vi "Create and Write Header.vi"(0 "reference in":refnum<class "RPC.lvclass">, 5 "error in (no error)":errorcluster) -> (7 "Nb Channels":i32, 9 "Total Nb Samples":i32, 11 "Scaling factors":dbl[](array[numeric]), 13 "Nb Groups":i32, 14 "reference out":refnum<class "RPC.lvclass">, 19 "error out":errorcluster)   [LabVIEW 2022 SP3, in "RPC.lvclass"]
uses:
  RPC.lvclass
  API/GSwFormDSP_class/GSwFormDSP.lvclass
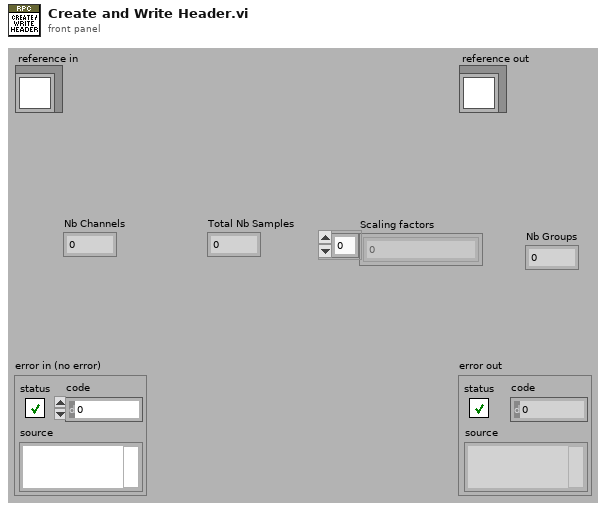
[diagram p1: front panel]
types:
  T1 = typedef "RPC.lvclass/ObjectAttributes.ctl" = cluster{"File Refnum":refnum<file>, "File total size":i32, "Offset from start of file":i32, "Time Type":enum16{"Response", "Drive"}, "Full Scale":dbl[unit], "New Time Data Obj?":bool, "Header":cluster{"Num Header":i32, "Num Parameter":i32, "Nb Channels":i32, "dT":dbl, "Number of Groups":i32, "Group size":i32, "Units":string[], "Names":string[], "Sensitivity":dbl[], "Complete header":string[]}, "Time Data":refnum<class "GSwFormDSP.lvclass">}
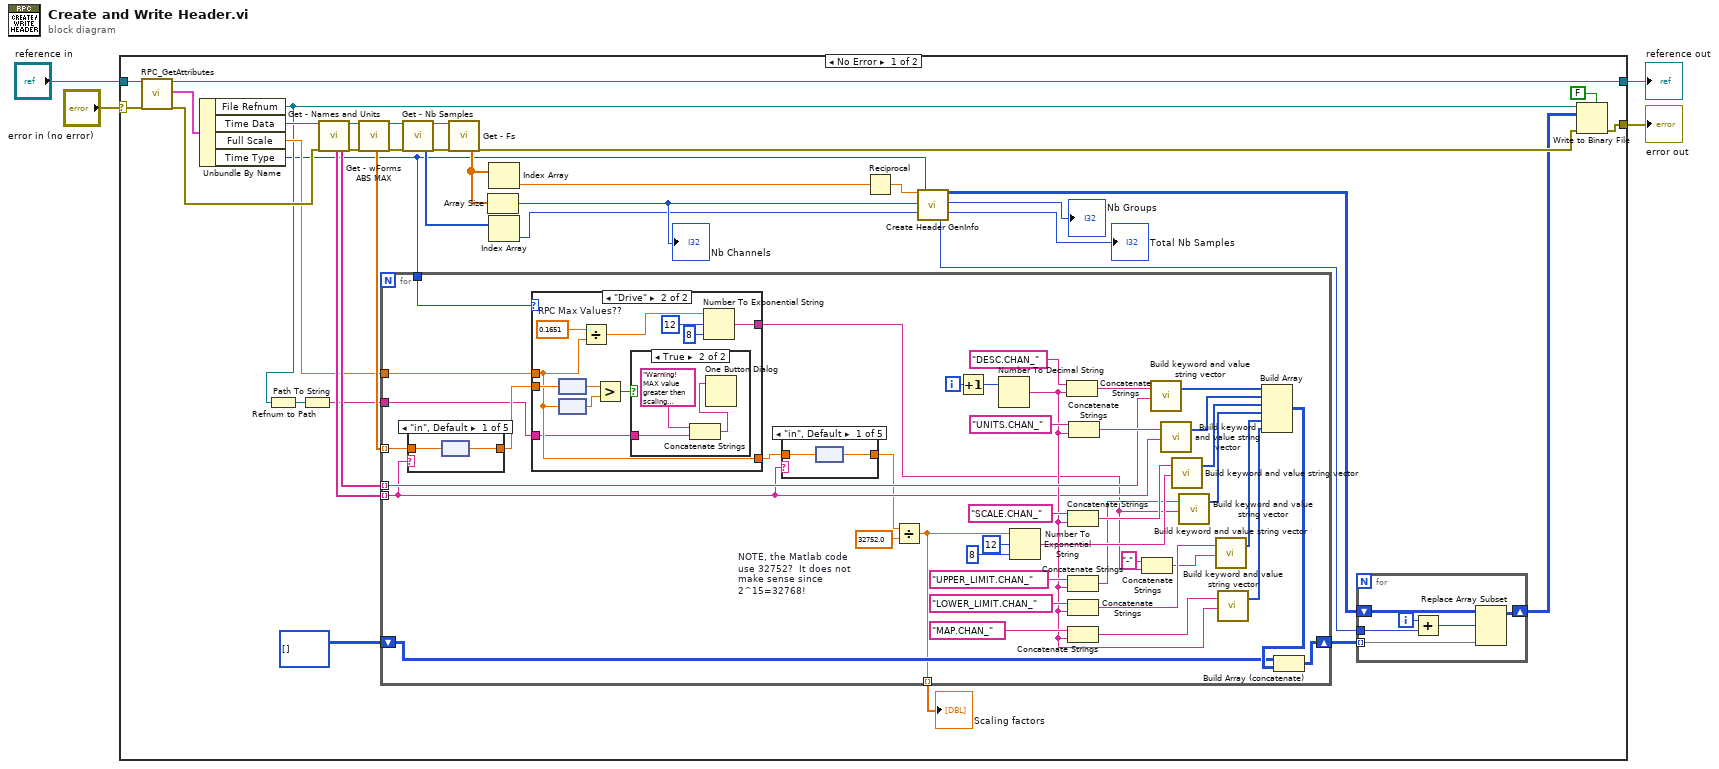
[diagram p0: block diagram]
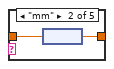
[diagram p2: hidden frame]
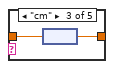
[diagram p3: hidden frame]
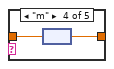
[diagram p4: hidden frame]
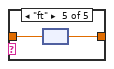
[diagram p5: hidden frame]
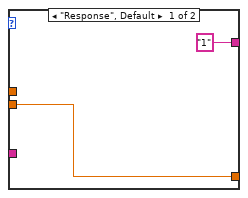
[diagram p6: hidden frame]
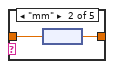
[diagram p8: hidden frame]
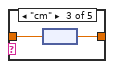
[diagram p9: hidden frame]
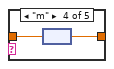
[diagram p10: hidden frame]
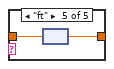
[diagram p11: hidden frame]
diagram:
  n1 = case shown="No Error" "error in (no error)" {
    selector: "error in (no error)" -> [w41 w126]
    tunnel: [w16 w126] -> w3
    tunnel: [w40 w125] -> w1
    tunnel: "reference in" -> [w38 w125]
    frame No Error {
      n2 = call "RPC_GetAttributes.vi"("reference in"=w38, "error in (no error)"=w41) -> ("reference out"=w40:refnum<class "RPC.lvclass">, "attributes"=w39:T1, "error out"=w10:errorcluster)  [unwired: 14 in, 1 out]
      n3 = Unbundle By Name(w39) -> ("File Refnum"=w7:refnum<file>, "Time Data"=w32:refnum<class "GSwFormDSP.lvclass">, "Full Scale"=w9:dbl[unit], "Time Type"=w5:enum16{"Response", "Drive"})
      n4 = Refnum to Path(1:w7) -> (0:w8:path)
      n5 = Path To String(path=w8) -> (string=w6:string)
      n6 = call-dynamic "Get - Names and Units.vi"("reference in"=w32, "error in (no error)"=w10) -> ("Signal Units"=w29:string[], "Signal Names"=w30:string[], "reference out"=w31:refnum<class "GSwFormDSP.lvclass">, "error out"=w28:errorcluster)  [unwired: 13 in, 1 out]
      n7 = call-dynamic "Get - wForms ABS MAX.vi"("reference in"=w31, "error in (no error)"=w28) -> ("ABS Max's"=w27:dbl[], "reference in"=w26:refnum<class "GSwFormDSP.lvclass">, "error out"=w25:errorcluster)  [unwired: 15 in]
      n8 = for {
        shift-right: [w64] -> w19
        shift-left: u8[][] [] -> [w63]
        tunnel: [w61] -> w22 mode=indexing
        tunnel: w27 -> [w58] mode=indexing
        tunnel: w30 -> [w60] mode=indexing
        tunnel: w29 -> [w53] mode=indexing
        tunnel: w5 -> [w57]
        tunnel: w9 -> [w56]
        tunnel: w6 -> [w54]
        i -> [w87]
        w88 = 32752.0  # NOTE, the Matlab code use 32752?  It does not make sense since 2^15=32768!
        n9 = case shown="\"in\", Default" w53 {
          tunnel: w58 -> [w116 w118 w120 w122 w124]
          tunnel: [w115 w117 w119 w121 w123] -> w55
          frame "in", Default {
            n10 = node(w116) -> (w115:dbl[unit])
          }
          frame "mm" {
            n11 = node(w118) -> (w117:dbl[unit])
          }
          frame "cm" {
            n12 = node(w120) -> (w119:dbl[unit])
          }
          frame "m" {
            n13 = node(w122) -> (w121:dbl[unit])
          }
          frame "ft" {
            n14 = node(w124) -> (w123:dbl[unit])
          }
        }
        n15 = case shown="\"Drive\"" w57 {
          tunnel: w55 -> [w99 w104]
          tunnel: [w99 w102] -> w52
          tunnel: w56 -> [_ w102]
          tunnel: ["1" w106] -> w49
          tunnel: w54 -> [_ w101]
          frame "Response", Default {
          }
          frame "Drive" {
            w110 = dbl[unit] 0.1651  # RPC Max Values??
            n16 = node(w104) -> (w103:dbl)
            n17 = node(w102) -> (w105:dbl)
            n18 = Divide(x=w110, y=w102) -> (x/y=w109:dbl)
            n19 = Greater?(x=w103, y=w105) -> (0:w111:bool)
            n20 = case shown="True" w111 {
              tunnel: w101 -> [_ w113]
              frame False {
              }
              frame True {
                n21 = Concatenate Strings("Warning! MAX value greater then scaling factor?\n", w113) -> (w112:string)
                n22 = One Button Dialog(message=w112) -> ()  [unwired: 1 in, 1 out]
              }
            }
            n23 = Number To Exponential String(number=w109, precision (6)=i16 8, 3:i16 12 ("width (-)")) -> (E-format string=w106:string)  [unwired: 1 out]
          }
        }
        n24 = case shown="\"in\", Default" w53 {
          tunnel: w52 -> [w90 w92 w94 w96 w98]
          tunnel: [w89 w91 w93 w95 w97] -> w51
          frame "in", Default {
            n25 = node(w90) -> (w89:dbl)
          }
          frame "mm" {
            n26 = node(w92) -> (w91:dbl)
          }
          frame "cm" {
            n27 = node(w94) -> (w93:dbl)
          }
          frame "m" {
            n28 = node(w96) -> (w95:dbl)
          }
          frame "ft" {
            n29 = node(w98) -> (w97:dbl)
          }
        }
        n30 = Divide(x=w51, y=w88) -> (x/y=w61:dbl)
        n31 = Increment(x=w87) -> (x+1=w62:i32)
        n32 = Number To Decimal String(number=w62) -> (decimal integer string=w59:string)  [unwired: 1 out]
        n33 = Number To Exponential String(number=w61, precision (6)=i16 8, 3:i16 12 ("width (-)")) -> (E-format string=w78:string)  [unwired: 1 out]
        n34 = Concatenate Strings("DESC.CHAN_", w59) -> (w85:string)
        n35 = Concatenate Strings("SCALE.CHAN_", w59) -> (w81:string)
        n36 = Concatenate Strings("UPPER_LIMIT.CHAN_", w59) -> (w76:string)
        n37 = Concatenate Strings("LOWER_LIMIT.CHAN_", w59) -> (w74:string)
        n38 = Concatenate Strings("MAP.CHAN_", w59) -> (w72:string)
        n39 = Concatenate Strings("UNITS.CHAN_", w59) -> (w83:string)
        n40 = Concatenate Strings("-", w49) -> (w48:string)
        n41 = call "Build keyword and value string vector.vi"("Keywords"=w85, "Values"=w60) -> ("Keywords & Values in 128 Bytes vector"=w71:u8[])  [unwired: 17 in]
        n42 = call "Build keyword and value string vector.vi"("Keywords"=w83, "Values"=w53) -> ("Keywords & Values in 128 Bytes vector"=w70:u8[])  [unwired: 17 in]
        n43 = call "Build keyword and value string vector.vi"("Keywords"=w81, "Values"=w78) -> ("Keywords & Values in 128 Bytes vector"=w69:u8[])  [unwired: 17 in]
        n44 = call "Build keyword and value string vector.vi"("Keywords"=w76, "Values"=w49) -> ("Keywords & Values in 128 Bytes vector"=w68:u8[])  [unwired: 17 in]
        n45 = call "Build keyword and value string vector.vi"("Keywords"=w74, "Values"=w48) -> ("Keywords & Values in 128 Bytes vector"=w67:u8[])  [unwired: 17 in]
        n46 = call "Build keyword and value string vector.vi"("Keywords"=w72, "Values"=w59) -> ("Keywords & Values in 128 Bytes vector"=w66:u8[])  [unwired: 17 in]
        n47 = Build Array(w71, w70, w69, w68, w67, w66) -> (w65:u8[][])
        n48 = Build Array (concatenate)(w63, w65) -> (w64:u8[][])
      }
      "Scaling factors" <- w22
      n49 = call "Get - Nb Samples.vi"("reference in"=w26, "error in (no error)"=w25) -> ("Signals Nb Samples"=w24:i32[], "reference in"=w21:refnum<class "GSwFormDSP.lvclass">, "error out"=w20:errorcluster)  [unwired: 14 in, 1 out]
      n50 = call-dynamic "Get - Fs.vi"("reference in"=w21, "error in (no error)"=w20) -> ("Signals Fs"=w35:dbl[], "error out"=w15:errorcluster)  [unwired: 14 in, 2 out]
      n51 = Array Size(array=w35) -> (size(s)=w34:i32)
      "Nb Channels" <- w34
      n52 = Index Array(array=w35) -> (element=w37:dbl)  [unwired: 1 in]
      n53 = Index Array(array=w24) -> (element=w23:i32)  [unwired: 1 in]
      n54 = Reciprocal(x=w37) -> (1/x=w36:dbl)
      n55 = call "Create Header GenInfo.vi"("dT"=w36, "Nb Channels"=w34, "Nb Samples"=w23, "Time Type"=w5) -> ("First X General parameters"=w11:i32, "Binary Header Info"=w18:u8[][], "Nb Groups"=→"Nb Groups":i32, "Total Nb Samples"=→"Total Nb Samples":i32)  [unwired: 12 in]
      n56 = for {
        shift-right: [w46] -> w14
        shift-left: w18 -> [w47]
        tunnel: w19 -> [w43] mode=indexing
        tunnel: w11 -> [w42]
        i -> [w45]
        n57 = Add(x=w45, y=w42) -> (x+y=w44:i32)
        n58 = Replace Array Subset(array=w47, new element=w43, index (row)=w44) -> (w46:u8[][])  [unwired: 1 in]
      }
      n59 = Write to Binary File(file (use dialog)=w7, data=w14, error in=w15, 5:FALSE ("prepend array or string size? (T)")) -> (error out=w16:errorcluster)  [unwired: 4 out]
    }
    frame Error {
    }
  }
  "error out" <- w3
  "reference out" <- w1
